vi "FOCUS_V42.vi"(9 "X-pixels":sgl=256.0, 11 "Run":bool) -> (0 "Retrace pixels":sgl, 10 "Pixel Clock (Hz)":sgl)   [LabVIEW 2010] (continued)
                frame 2 {
                  # "line scan FScope"
                  n3345 = local read "LS X/Y"() -> (w6474:bool)
                  n3346 = case shown="True" w6474 {
                    tunnel: [w6512 w6513] -> w6475
                    frame False {
                      n3347 = local read "Y dim"() -> (w6512:sgl)
                    }
                    frame True {
                      n3348 = local read "X dim"() -> (w6513:sgl)
                    }
                  }
                  n3349 = Initialize Array(u32 0 ("element"), w6475) -> (w6476:u32[])
                  n3350 = Unbundle By Name(w6496) -> ("status"=w6494:bool)
                  n3351 = Unbundle By Name(w6492) -> ("status"=w6491:bool)
                  n3352 = Unbundle By Name(w6495) -> ("status"=w6493:bool)
                  n3353 = while {
                    tunnel: w6505 -> [w6585]
                    tunnel: w6504 -> [w6584]
                    tunnel: [w6583] -> w6503
                    tunnel: [w6575] -> w6502
                    shift-right: [w6523] -> w6472
                    shift-left: w6497 -> [w6535]
                    shift-right: [w6525] -> w6471
                    shift-left: w6497 -> [w6534]
                    tunnel: [w6579] -> w6499
                    tunnel: w6501 -> [w6579]
                    tunnel: [w6576] -> w6498
                    tunnel: w6500 -> [w6576]
                    shift-right: [w6529] -> _
                    shift-left: w6476 -> [w6518]
                    tunnel: w6494 -> [w6572]
                    tunnel: w6493 -> [w6577]
                    tunnel: w6491 -> [w6560]
                    shift-right: [w6566] -> _
                    shift-left: sgl 0.0 ("millisecond timer value") -> [w6569]
                    tunnel: w6489 -> [w6565]
                    tunnel: w6486 -> [w6563]
                    tunnel: [w6563] -> w6484
                    tunnel: [w6562] -> w6483
                    tunnel: w6485 -> [w6562]
                    tunnel: w6482 -> [w6528]
                    shift-right: [w6550] -> _
                    shift-left: w6480 -> [w6552]
                    shift-right: [w6548] -> _
                    shift-left: w6481 -> [w6549]
                    tunnel: w6474 -> [w6532]
                    tunnel: [w6521] -> w6473
                    i -> [w6527]
                    stop <- w6571 stop-if-true
                    n3354 = local read "ScaleCluster"() -> (w6558:T3)
                    n3355 = local read "Overlay Images"() -> (w6580:bool)
                    n3356 = Bundle("ScaleCluster"=w6558, "scans to read"=w6528) -> (w6550:T20)  [unwired: 1 in]
                    n3357 = call-poly <vilib>:"DAQmx Read (Digital 1D U32 1Chan NSamp).vi"("task/channels in"=w6585, "number of samples per channel"=w6528, "error in"=w6584) -> ("task out"=w6583:refnum<k21>, "data"=w6516:u32[], "error out"=w6575:errorcluster)  [unwired: 10 in]
                    n3358 = Not Equal?(x=w6550, y=w6552) -> (x != y?=w6551:bool)
                    n3359 = Multiply(x=u32 0 ("millisecond timer value"), y=w6518) -> (x*y=w6517:u32[])
                    n3360 = call-poly <vilib>:"Ramp Pattern.vi"("start"=0.0, "end"=6.283185307179586, "samples"=w6528) -> ("Ramp Pattern"=w6547:dbl[])  [unwired: 7 in, 1 out]
                    n3361 = case shown="False" w6551 {
                      tunnel: w6565 -> [_ w6591]
                      tunnel: [w6588 w6590] -> w6548
                      tunnel: w6550 -> [_ w6589]
                      tunnel: w6549 -> [w6588 _]
                      frame False {
                      }
                      frame True {
                        n3362 = call "ScaleScanlineFScope.vi"("Parameters"=w6591, "ScaleCluster"=w6589) -> ("ScanlineScaled"=w6590:dbl[][])
                      }
                    }
                    n3363 = Split Number(x=w6516) -> (hi(x)=w6582:u16[])  [unwired: 1 out]
                    n3364 = Sine(x=w6547) -> (sin(x)=w6545:dbl[])
                    n3365 = Split Number(x=w6582) -> (hi(x)=w6520:u8[], lo(x)=w6581:u8[])
                    n3366 = case shown="True" w6580 {
                      tunnel: w6520 -> [w6597 w6616]
                      tunnel: [w6597 w6599] -> w6533
                      tunnel: w6581 -> [w6596 w6618]
                      tunnel: [w6596 _] -> w6530
                      frame False {
                      }
                      frame True {
                        n3367 = To Word Integer(number=w6616) -> (16bit integer=w6617:i16[])
                        n3368 = Subtract(x=w6617, y=w6618) -> (x-y=w6598:i16[])
                        n3369 = Add(x=w6617, y=w6618) -> (x+y=w6612:i16[])
                        n3370 = Increment(x=w6612) -> (x+1=w6622:i16[])
                        n3371 = Divide(x=w6598, y=w6622) -> (x/y=w6621:dbl[])
                        n3372 = Absolute Value(x=w6598) -> (abs(x)=w6614:i16[])
                        n3373 = Multiply(x=w6621, y=u8 2) -> (x*y=w6619:dbl[])
                        n3374 = Round To Nearest(number=w6619) -> (nearest integer value=w6605:dbl[])
                        n3375 = Divide(x=w6614, y=2.0) -> (x/y=w6611:dbl[])
                        n3376 = Divide(x=w6612, y=2.0) -> (x/y=w6610:dbl[])
                        n3377 = Add(x=w6611, y=w6610) -> (x+y=w6608:dbl[])
                        n3378 = Divide(x=w6608, y=5.0) -> (x/y=w6607:dbl[])
                        n3379 = Round To Nearest(number=w6607) -> (nearest integer value=w6606:dbl[])
                        n3380 = Multiply(x=5.0 ("y"), y=w6606) -> (x*y=w6604:dbl[])
                        n3381 = Add(x=w6605, y=w6604) -> (x+y=w6603:dbl[])
                        n3382 = Subtract(x=w6603, y=2.0) -> (x-y=w6600:dbl[])
                        n3383 = To Unsigned Byte Integer(number=w6600) -> (unsigned 8bit integer=w6599:u8[])
                      }
                    }
                    n3384 = Add(x=w6545, y=sgl 2.0 ("millisecond timer value")) -> (x+y=w6540:dbl[])
                    n3385 = Divide(x=u32 4294967295 ("millisecond timer value"), y=sgl 3.0) -> (x/y=w6541:sgl)
                    n3386 = Array Subset(array=w6548, index (col)=w6569, length (col)=w6528) -> (w6531:dbl[][])  [unwired: 2 in]
                    n3387 = Multiply(x=w6541, y=w6540) -> (x*y=w6539:dbl[])
                    n3388 = To Unsigned Long Integer(number=w6539) -> ()  [unwired: 1 out]
                    n3389 = Index Array(array=w6548, index (row)=0) -> (element=w6556:dbl[])  [unwired: 1 in]
                    n3390 = Array Size(array=w6556) -> (size(s)=w6554:i32)
                    n3391 = Divide(x=w6554, y=2) -> (x/y=w6553:dbl)
                    n3392 = Add(x=w6569, y=w6528) -> (x+y=w6567:dbl)
                    n3393 = local read "LS X/Y"() -> (w6537:bool)
                    n3394 = Greater Or Equal?(x=w6567, y=w6553) -> (x >= y?=w6568:bool)
                    n3395 = case shown="False" w6537 {
                      tunnel: [w6586 w6587] -> w6536
                      frame False {
                        n3396 = local read "X dim"() -> (w6586:sgl)
                      }
                      frame True {
                        n3397 = local read "Y dim"() -> (w6587:sgl)
                      }
                    }
                    n3398 = case shown="True" w6568 {
                      tunnel: w6567 -> [w6592 w6595]
                      tunnel: [w6592 w6593] -> w6566
                      tunnel: w6553 -> [_ w6594]
                      frame False {
                      }
                      frame True {
                        n3399 = Subtract(x=w6595, y=w6594) -> (x-y=w6593:dbl)
                      }
                    }
                    n3400 = Decrement(x=w6536) -> (x-1=w6561:sgl)
                    n3401 = Equal?(x=w6561, y=w6527) -> (x = y?=w6559:bool)
                    n3402 = call "AverageImageLSFScope.vi"("Index"=w6527, "ScanLineFScope"=w6531, "DataImage2"=w6530, "DataImage1"=w6533, "Image2Array"=w6534, "LS X/Y"=w6532, "Image1Array"=w6535, "HitsArrayLS"=w6517) -> ("Image2Arraynew"=w6525:u8[][], "Image1Arraynew"=w6523:u8[][], "HitsArrayLSnew"=w6529:u32[])
                    n3403 = local read "X dim"() -> (w6526:sgl)
                    n3404 = Build Array(w6529) -> (w6515:u32[][])
                    n3405 = Subtract(x=w6527, y=w6526) -> (x-y=w6521:sgl)
                    n3406 = Transpose 2D Array(2D array=w6515) -> (transposed array=w6514:u32[][])
                    n3407 = Array Subset(array=w6525, index (col)=w6521, length (col)=w6526) -> (w6524:u8[][])  [unwired: 2 in]
                    n3408 = local write "Hit Graph"(w6514) -> ()
                    n3409 = Array Subset(array=w6523, index (col)=w6521) -> (w6522:u8[][])  [unwired: 3 in]
                    n3410 = local write "Image 2"(w6524) -> ()
                    n3411 = local write "Image 1"(w6522) -> ()
                    n3412 = Unbundle By Name(w6562) -> ("status"=w6564:bool)
                    n3413 = Unbundle By Name(w6575) -> ("status"=w6573:bool)
                    n3414 = Unbundle By Name(w6576) -> ("status"=w6574:bool)
                    n3415 = local read "stop 2"() -> (w6578:bool)
                    n3416 = local read "End experiment"() -> (w6570:bool)
                    n3417 = Compound Arithmetic op=OR(w6578, w6577, w6574, w6573, w6572, w6564, w6559, w6560, w6570) -> (w6571:bool)
                  }
                }
              }
            }
          }
          "ScanLineLength" <- w3421
          "ZSinLength" <- w3420
          "DataOffset" <- w3419
          n3418 = Round Toward +Infinity(x=w3376) -> (ceil(x): smallest int >= x=w3378:sgl)
          n3419 = property on="ImageSlide" class="Slide (strict)"("Scale.Range:Minimum"=0.0, "Scale.Range:Maximum"=w3376) -> ()  [unwired: 2 in, 2 out]
          n3420 = local write "ImageSlide"(w3378) -> ()
          n3421 = Equal?(x=w3402, y=w3401) -> (x = y?=w3390:bool)
          n3422 = Multiply(x=sgl 1000.0, y="Time interval [s]") -> (x*y=w3311:sgl)
          n3423 = Not(x=w3399) -> (.not. x?=w3389:bool)
          n3424 = local read "Zsin3D"() -> (w3321:sgl[])
          n3425 = Subtract(x=w3311, y=w3363) -> ()  [unwired: 1 out]
          n3426 = In Range and Coerce(upper limit=w3311, x=w3311, lower limit=sgl 0.0) -> (coerced(x)=w3361:sgl)  [unwired: 1 out]
          n3427 = Array Size(array=w3338) -> (size(s)=w3337:i32[])
          n3428 = Array Size(array=w3335) -> (size(s)=w3336:i32[])
          n3429 = Or(x=w3389, y=w3390) -> (x .or. y?=w3391:bool)
          n3430 = local read "frame/line indicator"() -> (w3324:u16)
          n3431 = Multiply Array Elements(1:w3337) -> (0:w3334:i32)
          n3432 = Multiply Array Elements(1:w3336) -> (0:w3333:i32)
          n3433 = Unbundle(w3342) -> ("Output: VISA session OUT"=w3346:refnum<visa-resource-name>, "Error cluster"=w3345:errorcluster)
          n3434 = Index Array(array=w3320, index (row)=0 ("disabled index (col)")) -> (element=w3315:sgl[])  [unwired: 1 in]
          n3435 = Index Array(array=w3320, index (row)=1 ("disabled index (col)")) -> (element=w3314:sgl[])  [unwired: 1 in]
          n3436 = Add(x=w3334, y=w3333) -> (x+y=w3332:i32)
          "DataLength" <- w3332
          n3437 = property class="Serial Instr"(reference=w3346, error in=w3345) -> (reference out=w3347:refnum<visa-resource-name>, error out=w3348:errorcluster, "Serial Settings:Number of Bytes at Serial Port"=w3349:u32)
          n3438 = Interleave 1D Arrays(w3315, w3314, w3321) -> (w3319:sgl[])
          n3439 = local read "Positions"() -> (w3313:sgl[])
          n3440 = Greater Than 0?(x=w3324) -> (x > 0?=w3323:bool)
          n3441 = Greater Or Equal?(x=w3324, y=u16 3) -> (x >= y?=w3326:bool)
          n3442 = Array Size(array=w3319) -> (size(s)=w3318:i32)
          n3443 = property on="Property Node" class="VI"() -> ("VI Path"=w3327:path)  [unwired: 2 in, 2 out]
          n3444 = Build Array (concatenate)(w3318, w3319, w3313) -> (w3312:sgl[])
          n3445 = VISA Read(VISA resource name=w3347, byte count=w3349, error in (no error)=w3348) -> (VISA resource name out=w3343:refnum<visa-resource-name>, error out=w3344:errorcluster)  [unwired: 2 out]
          n3446 = case shown="True" w3323 {
            tunnel: w3326 -> [_ w3444]
            tunnel: w3327 -> [_ w3443]
            tunnel: w3322 -> [_ w3442]
            tunnel: w3312 -> [_ w3441]
            frame False {
            }
            frame True {
              n3447 = case shown="True" "Autosave" {
                tunnel: w3444 -> [_ w3450]
                tunnel: w3442 -> [_ w3448]
                tunnel: w3443 -> [_ w3447]
                tunnel: w3441 -> [_ w3446]
                frame False {
                }
                frame True {
                  n3448 = local read "FilePath"() -> (w3452:path)
                  n3449 = local read "BaseFilename"() -> (w3451:string)
                  n3450 = Bundle("BaseFilename"=w3451, "FilePath"=w3452, "Autoincrement\nFilename"=TRUE ("Autoincrement\nFilename"), w3450) -> (w3449:T35)  [unwired: 1 in]
                  n3451 = call "SavenewFOCUS.vi"("source path"=w3447, "Header"=w3448, "Positions"=w3446, "Parameters"=w3449) -> ("Data directory out"=w3454:path, "name"=w3456:string, "basename out"=w3455:string)
                  n3452 = local write "Save?"(TRUE ("Save?")) -> ()
                  n3453 = local write "BaseFilename"(w3455) -> ()
                  n3454 = local write "FilePath"(w3454) -> ()
                  n3455 = local write "Filename"(w3456) -> ()
                }
              }
            }
          }
          n3456 = local read "Sutter scale x"() -> (w3300:sgl)
          n3457 = local read "Sutter scale y"() -> (w3299:sgl)
          n3458 = local read "Sutter scale z"() -> (w3298:sgl)
          n3459 = Bundle("Output: VISA session OUT"=w3343, "error out"=w3344) -> (w3341:T36)  [unwired: 1 in]
          n3460 = call "VISA MP-285 Get Position.vi"("Input: Duty Cluster"=w3341) -> ("Output: X axis (microns)"=w3357:dbl, "Output: Y axis (microns)"=w3356:dbl, "Output: Z axis (microns)"=w3355:dbl, "Output: Duty Cluster"=w3351:T18)
          n3461 = case shown="False" w3391 {
            tunnel: [w6681 w6705] -> w3383
            tunnel: w3351 -> [w6680 w6707]
            tunnel: [w6679 w6707] -> w3350
            tunnel: [w6678 w6704] -> w3397
            tunnel: w3395 -> [w6677 w6705]
            tunnel: w3394 -> [w6676 w6704]
            tunnel: w3386 -> [w6675 w6706]
            tunnel: w3393 -> [w6674 w6708]
            tunnel: [w6673 w6708] -> w3392
            tunnel: w3361 -> [w6672 _]
            tunnel: [w6671 w6706] -> w3385
            frame False {
              n3462 = local read "Number of frames"() -> (w6667:sgl)
              n3463 = flat-sequence {
                tunnel: w6672 -> [w6693]
                tunnel: [w6693] -> w6687
                tunnel: [w6689] -> w6686
                tunnel: [w6688] -> w6685
                tunnel: w6677 -> [w6691]
                tunnel: w6676 -> [w6690]
                tunnel: [w6700] -> w6684
                tunnel: [w6699] -> w6683
                tunnel: [w6698] -> w6682
                tunnel: w6687 -> [w6700]
                tunnel: w6686 -> [w6699]
                tunnel: w6685 -> [w6698]
                tunnel: w6675 -> [w6697]
                tunnel: w6674 -> [w6696]
                tunnel: [w6695] -> w6673
                tunnel: [w6694] -> w6671
                tunnel: [w6703] -> w6681
                tunnel: [w6702] -> w6678
                tunnel: w6684 -> [w6701]
                tunnel: w6683 -> [w6703]
                tunnel: w6682 -> [w6702]
                frame #0 {
                  w6692 = FALSE ("data")
                  n3464 = local write "Shutter open"(w6692) -> ()
                  n3465 = call-poly <vilib>:"DAQmx Write (Digital Bool 1Line 1Point).vi"("task/channels in"=w6691, "data"=w6692, "error in"=w6690) -> ("task out"=w6689:refnum<k21>, "error out"=w6688:errorcluster)  [unwired: 10 in, 1 out]
                }
                frame #1 {
                  n3466 = call <vilib>:"DAQmx Stop Task.vi"("task/channels in"=w6697, "error in"=w6696) -> ("task out"=w6694:refnum<k21>, "error out"=w6695:errorcluster)  [unwired: 12 in]
                }
                frame #2 {
                  n3467 = Wait (ms)(milliseconds to wait=w6701) -> ()  [unwired: 1 out]
                }
              }
              n3468 = local read "z-step (um)"() -> (w6669:sgl)
              n3469 = local read "Sutter scale z"() -> (w6665:sgl)
              n3470 = Decrement(x=w6667) -> (x-1=w6666:sgl)
              n3471 = Multiply(x=w6669, y=w6666) -> (x*y=w6668:sgl)
              n3472 = Negate(x=w6665) -> (-x=w6664:sgl)
              n3473 = Divide(x=w6668, y=w6664) -> (x/y=w6670:sgl)
              n3474 = call "VISA MP-285 Step.vi"("Input: Duty Cluster"=w6680, "Input: Delta Z axis (microns)"=w6670) -> ("Output: Duty Cluster"=w6679:T18)  [unwired: 2 in, 3 out]
            }
            frame True {
            }
          }
          n3475 = Multiply(x=w3357, y=w3300) -> (x*y=→"x-positionstop (um)":dbl)
          n3476 = Multiply(x=w3356, y=w3299) -> (x*y=→"y-positionstop (um)":dbl)
          n3477 = Multiply(x=w3355, y=w3298) -> (x*y=→"z-positionstop (um)":dbl)
          n3478 = case shown="True" w3399 {
            tunnel: "Number of stacks" -> [_ w6726]
            tunnel: [TRUE w6721] -> w3398
            tunnel: w3401 -> [_ w6725]
            frame False {
            }
            frame True {
              n3479 = local read "End experiment"() -> (w6724:bool)
              n3480 = Increment(x=w6725) -> (x+1=w6720:i32)
              "#" <- w6720
              "#" <- w6720
              n3481 = local read "stop 2"() -> (w6723:bool)
              n3482 = Equal?(x=w6726, y=w6720) -> (x = y?=w6722:bool)
              n3483 = Compound Arithmetic op=OR(w6723, w6724, w6722) -> (w6721:bool)
            }
          }
          n3484 = case shown="True" w3398 {
            tunnel: w3397 -> [w6710 w6713]
            tunnel: [w6710 w6712] -> w3396
            tunnel: w3383 -> [w6709 w6714]
            tunnel: [w6709 w6711] -> w3382
            frame False {
            }
            frame True {
              w6715 = FALSE ("data")
              w6716 = u8 0 ("Disabled")
              w6717 = FALSE
              # "Sort out controls"
              n3485 = local write "stop 2"(w6717) -> ()
              n3486 = local write "Run"(w6717) -> ()
              n3487 = property on="Scan format" class="Ring (strict)"("Disabled"=w6716) -> ()  [unwired: 2 in, 2 out]
              n3488 = property on="X-pixels" class="DigNum (strict)"("Disabled"=w6716) -> ()  [unwired: 2 in, 2 out]
              n3489 = property on="Y-lines" class="DigNum (strict)"("Disabled"=w6716) -> ()  [unwired: 2 in, 2 out]
              n3490 = local write "Shutter open"(w6715) -> ()
              n3491 = call-poly <vilib>:"DAQmx Write (Digital Bool 1Line 1Point).vi"("task/channels in"=w6714, "data"=w6715, "error in"=w6713) -> ("task out"=w6711:refnum<k21>, "error out"=w6712:errorcluster)  [unwired: 10 in, 1 out]
              n3492 = property on="line scan time (ms)" class="DigNum (strict)"("Disabled"=w6716) -> ()  [unwired: 2 in, 2 out]
              n3493 = property on="Rotation" class="Knob (strict)"("Disabled"=w6716) -> ()  [unwired: 2 in, 2 out]
              n3494 = property on="Zoom" class="Slide (strict)"("Disabled"=w6716) -> ()  [unwired: 2 in, 2 out]
              n3495 = property on="Run" class="Bool (strict)"("Visible"=TRUE) -> ()  [unwired: 2 in, 2 out]
              n3496 = property on="Measurement cursor check box" class="Bool (strict)"("Disabled"=w6716) -> ()  [unwired: 2 in, 2 out]
              n3497 = property on="View line\ncheck box" class="Bool (strict)"("Disabled"=w6716) -> ()  [unwired: 2 in, 2 out]
            }
          }
        }
      }
    }
    "Image1Array" <- w190
    "Image2Array" <- w189
    "Image3Array" <- w188
    "Image4Array" <- w187
    n3498 = case shown="True" w209 {
      tunnel: w216 -> [_ w346]
      tunnel: w215 -> [_ w345]
      frame False {
      }
      frame True {
        n3499 = call <vilib>:"DAQmx Clear Task.vi"("task in"=w345, "error in"=w346) -> ("error out"=w347:errorcluster)  [unwired: 13 in]
        n3500 = call <vilib>:"Simple Error Handler.vi"("error in (no error)"=w347) -> ()  [unwired: 4 in, 5 out]
      }
    }
    n3501 = stacked-sequence {
      tunnel: [w348] -> w251
      tunnel: w223 -> [_]
      frame #0 {
        n3502 = local read "AO/DIO Device"() -> (w348:tag)
      }
    }
    n3503 = local read "frame/line indicator"() -> (w254:u16)
    n3504 = local read "frame/line indicator"() -> (w257:u16)
    n3505 = Unbundle(w198) -> ("Output: VISA session OUT"=w202:refnum<visa-resource-name>, "Error cluster"=w201:errorcluster)
    n3506 = call <vilib>:"DAQmx Clear Task.vi"("task in"=w269, "error in"=w270) -> ("error out"=w268:errorcluster)  [unwired: 13 in]
    n3507 = call <vilib>:"DAQmx Clear Task.vi"("task in"=w273, "error in"=w272) -> ("error out"=w274:errorcluster)  [unwired: 13 in]
    n3508 = call <vilib>:"DAQmx Clear Task.vi"("task in"=w266, "error in"=w265) -> ("error out"=w264:errorcluster)  [unwired: 13 in]
    n3509 = property class="Serial Instr"(reference=w202, error in=w201) -> (reference out=w203:refnum<visa-resource-name>, error out=w204:errorcluster, "Serial Settings:Number of Bytes at Serial Port"=w205:u32)
    n3510 = call <vilib>:"Simple Error Handler.vi"("error in (no error)"=w274) -> ()  [unwired: 4 in, 5 out]
    n3511 = call <vilib>:"Simple Error Handler.vi"("error in (no error)"=w268) -> ()  [unwired: 4 in, 5 out]
    n3512 = call <vilib>:"DAQmx Clear Task.vi"("task in"=w267, "error in"=w264) -> ("error out"=w262:errorcluster)  [unwired: 13 in]
    n3513 = Equal?(x=w254, y=u16 4) -> (x = y?=w165:bool)
    n3514 = Concatenate Strings(tag "/" ("destination terminal"), w251) -> (w227:string)
    n3515 = Concatenate Strings(w227, tag "/PXI_Trig2" ("source terminal")) -> (w238:string)
    n3516 = Concatenate Strings(w227, tag "/PFI2" ("destination terminal")) -> (w240:string)
    n3517 = Concatenate Strings(w227, tag "/PXI_Trig2" ("destination terminal")) -> (w247:string)
    n3518 = Concatenate Strings(w227, tag "/10MHzRefClock" ("source terminal")) -> (w250:string)
    n3519 = Type Cast(type=tag "" ("destination terminal"), x=w238) -> (*(type *) &x=w236:tag)
    n3520 = Type Cast(type=tag "" ("destination terminal"), x=w240) -> (*(type *) &x=w235:tag)
    n3521 = Type Cast(type=tag "" ("destination terminal"), x=w247) -> (*(type *) &x=w243:tag)
    n3522 = Type Cast(type=tag "" ("destination terminal"), x=w250) -> (*(type *) &x=w244:tag)
    n3523 = call <vilib>:"DAQmx Disconnect Terminals.vi"("source terminal"=w244, "destination terminal"=w243, "error in"=w279) -> ("error out"=w280:errorcluster)  [unwired: 12 in]
    n3524 = Greater Or Equal?(x=w257, y=u16 3) -> (x >= y?=w255:bool)
    n3525 = call <vilib>:"Simple Error Handler.vi"("error in (no error)"=w262) -> ()  [unwired: 4 in, 5 out]
    n3526 = Or(x=w165, y=w163) -> (x .or. y?=w164:bool)
    n3527 = VISA Read(VISA resource name=w203, byte count=w205, error in (no error)=w204) -> (VISA resource name out=w199:refnum<visa-resource-name>, error out=w200:errorcluster)  [unwired: 2 out]
    n3528 = case shown="True" w255 {
      tunnel: w271 -> [_ w353]
      tunnel: w223 -> [_ w352]
      frame False {
      }
      frame True {
        n3529 = call <vilib>:"DAQmx Clear Task.vi"("task in"=w353, "error in"=w352) -> ("error out"=w354:errorcluster)  [unwired: 13 in]
        n3530 = call <vilib>:"Simple Error Handler.vi"("error in (no error)"=w354) -> ()  [unwired: 4 in, 5 out]
      }
    }
    n3531 = call <vilib>:"DAQmx Disconnect Terminals.vi"("source terminal"=w236, "destination terminal"=w235, "error in"=w280) -> ("error out"=w234:errorcluster)  [unwired: 12 in]
    n3532 = Concatenate Strings(w227, tag "/PFI5" ("destination terminal")) -> (w231:string)
    n3533 = case shown="False" w164 {
      tunnel: w293 -> [w351 _]
      tunnel: w292 -> [w350 _]
      frame False {
        n3534 = call <vilib>:"DAQmx Clear Task.vi"("task in"=w350, "error in"=w351) -> ("error out"=w349:errorcluster)  [unwired: 13 in]
        n3535 = call <vilib>:"Simple Error Handler.vi"("error in (no error)"=w349) -> ()  [unwired: 4 in, 5 out]
      }
      frame True {
      }
    }
    n3536 = Concatenate Strings(w227, tag "/ao/SampleClock" ("source terminal")) -> (w228:string)
    n3537 = Type Cast(type=tag "" ("destination terminal"), x=w231) -> (*(type *) &x=w226:tag)
    n3538 = Bundle("Output: VISA session OUT"=w199, "error out"=w200) -> (w161:T36)  [unwired: 1 in]
    n3539 = Type Cast(type=tag "" ("destination terminal"), x=w228) -> (*(type *) &x=w225:tag)
    n3540 = call <vilib>:"DAQmx Disconnect Terminals.vi"("source terminal"=w225, "destination terminal"=w226, "error in"=w234) -> ("error out"=w224:errorcluster)  [unwired: 12 in]
    n3541 = call <vilib>:"DAQmx Clear Task.vi"("task in"=w277, "error in"=w224) -> ("error out"=w278:errorcluster)  [unwired: 13 in]
    n3542 = call <vilib>:"Simple Error Handler.vi"("error in (no error)"=w278) -> ()  [unwired: 4 in, 5 out]
    "Line Clock" <- w297
    "Frame Clock" <- w261
    "Position Signals" <- w260
    "Scan Signals" <- w259
    "Data Input" <- w258
  }
  n3543 = flat-sequence {
    tunnel: [w6798] -> w6
    tunnel: w4 -> [_]
    frame #0 {
      w6801 = "L"  # Resolution (L or H)
      n3544 = Type Cast(type=" ", x="VISA Sutter MP-285") -> (*(type *) &x=w6806:string)
      n3545 = Reverse String(1:w6806) -> (0:w6805:string)
      n3546 = String Subset(string=w6805, offset (0)=0, length (rest)=1 ("length (rest)")) -> (substring=w6802:string)
      n3547 = Decimal String To Number(string=w6802) -> (number=w6809:i32)  [unwired: 2 in, 1 out]
      n3548 = local read "Sutter Speed [um/s]"() -> (w6797:i32)
      n3549 = call "VISA MP-285 InitNotRefresh.vi"("baud rate (9600)"=u32 9600, "Timeout (msec)"=u32 700, "Serial port # \n(COM1 - #1)!!!"=w6809) -> ("Output: Duty Cluster"=w6800:T18)  [unwired: 1 in]
      n3550 = call "VISA MP-285 GetSet Resolution.vi"("Input: Resolution - H/L"=w6801, "Input: Duty Cluster"=w6800) -> ("Output: Duty Cluster"=w6799:T18)  [unwired: 2 out]
      n3551 = Add(x=w6797, y=300) -> (x+y=w6795:i32)
      n3552 = call "VISA MP-285 GetSet Speed.vi"("Input: Duty Cluster"=w6799, "Input: Speed in microns/sec"=w6795) -> ("Output: Duty Cluster"=w6798:T18)  [unwired: 1 out]
    }
  }
  n3553 = call "VISA MP-285 Close.vi"("Input: Duty Cluster"=w5) -> ()  [unwired: 1 out]
  "Program Version" <- w87
